vi "Test.vi"() -> ()   [LabVIEW 2017]
uses:
  <vilib>/sound2/lvsound2.llb/Sampling Mode.ctl
  <vilib>/sound2/lvsound2.llb/Sound File Position.ctl
  <vilib>/sound2/lvsound2.llb/Sound File Info (path).vi
  <vilib>/sound2/lvsound2.llb/Sound File Read Open.vi
  <vilib>/sound2/lvsound2.llb/Sound File Read (DBL).vi
  <vilib>/sound2/lvsound2.llb/Sound Output Write (DBL).vi
panel:
  in  "stop":bool
  in  "path":path
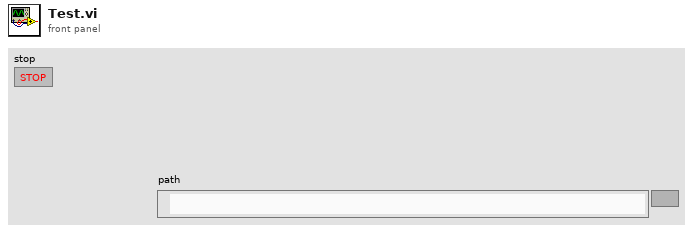
[diagram p1: front panel]
types:
  T1 = typedef "Sampling Mode.ctl" = i32
  T2 = typedef "Sound Data Format.ctl" = cluster{"sample rate (S/s)":dbl, "number of channels":i32, "bits per sample":i32}
  T3 = typedef "Sound File Refnum.ctl" = refnum<file>
  T4 = typedef "Sound Output Task ID.ctl" = u32
  T5 = typedef "Sound File Position.ctl" = u16
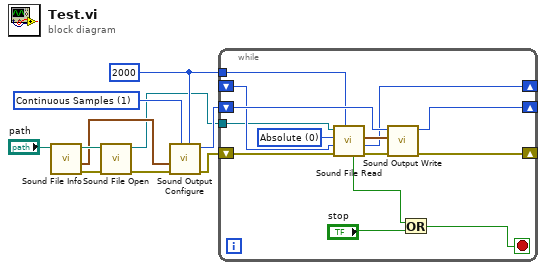
[diagram p0: block diagram]
diagram:
  w2 = 2000 ("number of samples/ch")
  w8 = T1 1 items=["Finite Samples", "Continuous Samples"] ("sample mode")
  n1 = call-poly <vilib>:"Sound File Info.vi"("path"="path") -> ("error out"=w6:errorcluster, "sound format"=w7:T2, "path out"=w9:path)  [unwired: 7 in, 1 out]
  n2 = call-poly <vilib>:"Sound File Open.vi"("error in (no error)"=w6, "path"=w9) -> ("error out"=w5:errorcluster, "sound file refnum"=w1:T3)  [unwired: 8 in]
  n3 = call <vilib>:"Sound Output Configure.vi"("number of samples/ch"=w2, "sample mode"=w8, "error in (no error)"=w5, "sound format"=w7) -> ("error out"=w4:errorcluster, "task ID"=w3:T4)  [unwired: 6 in]
  n4 = while {
    shift-right: [w22] -> _
    shift-left: w4 -> [w24]
    shift-right: [w19] -> _
    shift-left: w3 -> [w20]
    shift-right: [w18] -> _
    shift-left: _ -> [w16]
    tunnel: w2 -> [w17]
    tunnel: w1 -> [w15]
    stop <- w12 stop-if-true
    w14 = T5 0 items=["Absolute"=0, "Relative"=2] ("position mode")
    n5 = call-poly <vilib>:"Sound File Read.vi"("number of samples/ch (-1: all)"=w17, "error in (no error)"=w24, "position offset"=w16, "position mode"=w14, "sound file refnum"=w15) -> ("error out"=w23:errorcluster, "offset"=w18:i32, "data"=w21:waveform(dbl)[], "end of file?"=w11:bool)  [unwired: 2 in, 1 out]
    n6 = call-poly <vilib>:"Sound Output Write.vi"("error in (no error)"=w23, "data"=w21, "task ID"=w20) -> ("error out"=w22:errorcluster, "task ID out"=w19:T4)  [unwired: 7 in]
    n7 = Or(x=w11, y="stop") -> (x .or. y?=w12:bool)
  }
